vi "PZT feedback.vi"(8 "error in":errorcluster, 9 "PZT step":i16, 10 "fine_approach setpoint":dbl, 11 "Coarse Approach.lvclass":refnum<class "Coarse Approach.lvclass">) -> (0 "error out":errorcluster, 1 "Amplitude (V rms)":dbl, 2 "Z Voltage out":i16(slide) scale=32767.0..-32768.0, 3 "Coarse Approach.lvclass":refnum<class "Coarse Approach.lvclass">)   [LabVIEW 2020, in "Coarse Approach.lvclass"]
uses:
  Coarse Approach.lvclass
  Coarse Approach.lvclass/Coarse Approach.ctl
  Lock-In Amplifier/Lock-In Amplifier.lvclass
  PI P123.01 & PiezoDrive TD250 & NI USB 7855R/PI P123.01 & PiezoDrive TD250 & NI USB 7855R.lvclass
  PZT/PZT.lvclass
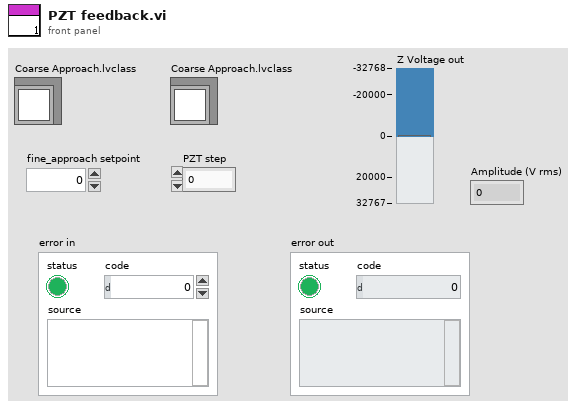
[diagram p1: front panel]
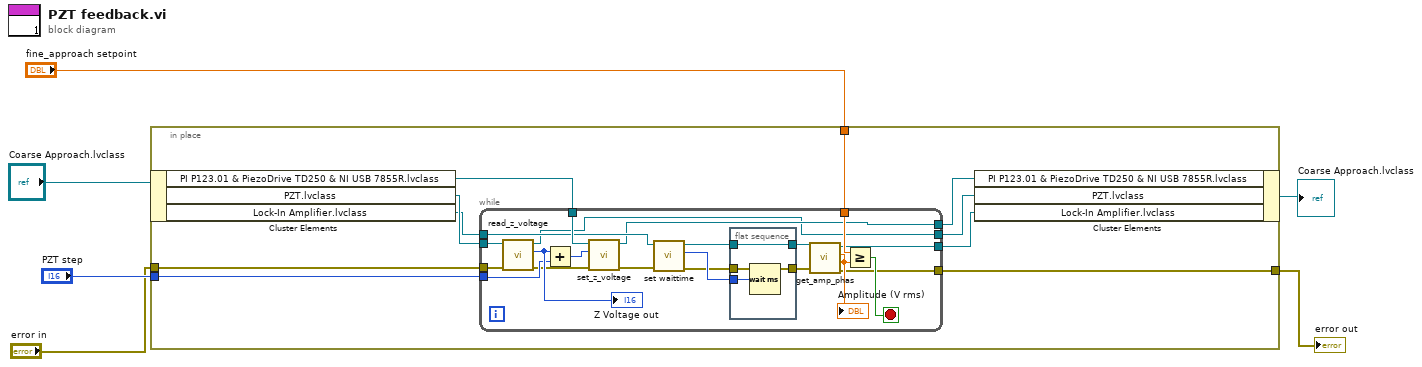
[diagram p0: block diagram]
diagram:
  n1 = in-place {
    in-place-border: "PZT step" -> [w14]
    in-place-border: "error in" -> [w13]
    in-place-border: "fine_approach setpoint" -> [w11]
    in-place-border: [w7] -> w2
    n2 = in-place-cluster #1("Coarse Approach.lvclass") -> ("PI P123.01 & PiezoDrive TD250 & NI USB 7855R.lvclass"=w15:refnum<class "PI P123.01 & PiezoDrive TD250 & NI USB 7855R.lvclass">, "PZT.lvclass"=w16:refnum<class "PZT.lvclass">, "Lock-In Amplifier.lvclass"=w12:refnum<class "Lock-In Amplifier.lvclass">)
    n3 = while {
      tunnel: w16 -> [w37]
      tunnel: w15 -> [w36]
      tunnel: w14 -> [w33]
      tunnel: w13 -> [w32]
      tunnel: w12 -> [w30]
      tunnel: w11 -> [w23]
      tunnel: [w20] -> w10
      tunnel: [w19] -> w9
      tunnel: [w18] -> w8
      tunnel: [w17] -> w7
      stop <- w21 stop-if-true
      n4 = call "read_z_voltage.vi"("error in"=w32, "PZT in"=w37) -> ("error out"=w31:errorcluster, "Z Voltage out"=w34:i16, "PZT out"=w19:refnum<class "PZT.lvclass">)  [unwired: 7 in]
      "Z Voltage out" <- w34
      n5 = Add(x=w34, y=w33) -> (x+y=w35:i16)
      n6 = call "set_z_voltage.vi"("error in (no error)"=w31, "Z Voltage (V)"=w35, "PI P123.01 & PiezoDrive TD250 & NI USB 7855R in"=w36) -> ("error out"=w27:errorcluster, "PI P123.01 & PiezoDrive TD250 & NI USB 7855R out"=w20:refnum<class "PI P123.01 & PiezoDrive TD250 & NI USB 7855R.lvclass">)  [unwired: 7 in]
      n7 = call "set waittime.vi"("error in"=w27, "Lock-In Amplifier"=w30) -> ("error out"=w26:errorcluster, "Wait time"=w29:u32, "Lock-In Amplifier"=w28:refnum<class "Lock-In Amplifier.lvclass">)  [unwired: 7 in]
      n8 = flat-sequence {
        tunnel: w29 -> [w40]
        tunnel: w28 -> [w39]
        tunnel: [w39] -> w25
        tunnel: w26 -> [w38]
        tunnel: [w38] -> w24
        frame #0 {
          n9 = Wait (ms)(milliseconds to wait=w40) -> ()  [unwired: 1 out]
        }
      }
      n10 = call-dynamic "get_amp_phas.vi"("error in (no error)"=w24, "Lock-In Amplifier in"=w25) -> ("error out"=w17:errorcluster, "Amplitude (V rms)"=w22:dbl, "Lock-In Amplifier out"=w18:refnum<class "Lock-In Amplifier.lvclass">)  [unwired: 6 in, 1 out]
      "Amplitude (V rms)" <- w22
      n11 = Greater Or Equal?(x=w23, y=w22) -> (x >= y?=w21:bool)
    }
    n12 = in-place-cluster #1("PI P123.01 & PiezoDrive TD250 & NI USB 7855R.lvclass"=w10, "PZT.lvclass"=w9, "Lock-In Amplifier.lvclass"=w8) -> (→"Coarse Approach.lvclass":refnum<class "Coarse Approach.lvclass">)
  }
  "error out" <- w2
